vi "Custom File Dialog.vi"(8 "error in (no error)":errorcluster) -> (0 "error out":errorcluster, 2 "path out":path)   [LabVIEW 2024, in "ImportExport.lvlib"]
uses:
  ImportExport.lvlib
panel:
  in  "OK Button":bool
  in  "Select the file path for your configuration.":path
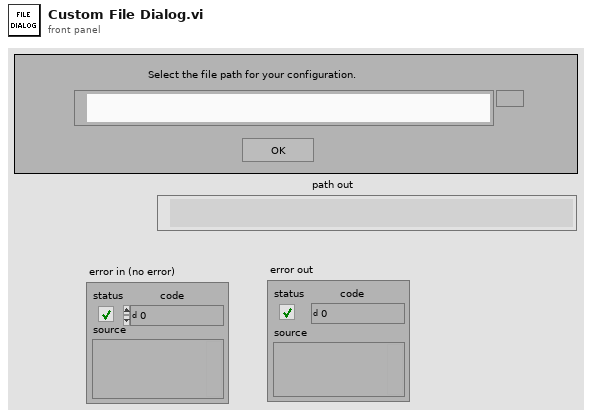
[diagram p1: front panel]
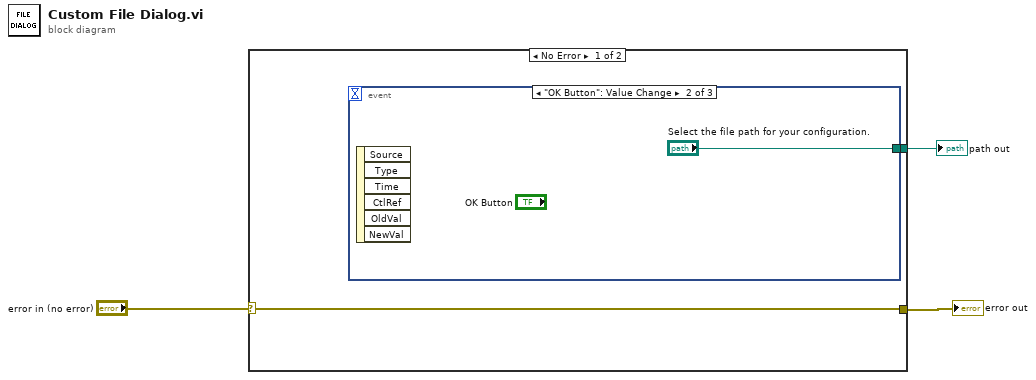
[diagram p0: block diagram]
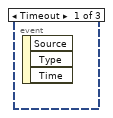
[diagram p2: hidden frame]
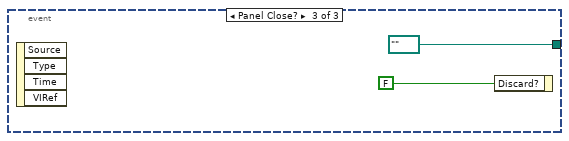
[diagram p3: hidden frame]
diagram:
  n1 = case shown="No Error" "error in (no error)" {
    selector: "error in (no error)" -> [w5 w9]
    tunnel: [w5 w9] -> w2
    tunnel: [w4 _] -> w1
    frame No Error {
      n2 = event shown="[1] \"OK Button\": Value Change" {
        selector: _ -> [_ _ _]
        dyn-events: _ -> [_ _ _]
        timeout: _ -> [_ _ _]
        tunnel: [_ "Select the file path for your configuration." path "" ("Folder path to export")] -> w4
        event Timeout {
          n3 = event-data() -> ()  [unwired: 1 in, 3 out]
        }
        event "OK Button": Value Change {
          n4 = event-data() -> ()  [unwired: 1 in, 6 out]
        }
        event Panel Close? {
          n5 = event-data() -> ()  [unwired: 1 in, 4 out]
          n6 = event-data("Discard?"=FALSE) -> ()  [unwired: 1 in, 1 out]
        }
      }
    }
    frame Error {
    }
  }
  "path out" <- w1
  "error out" <- w2
